vi "Filter_On_Start.vi"(10 "Num In":dbl[](array[numeric]), 11 "Denom In":dbl[](array[numeric])) -> (2 "Num out":dbl[](array[numeric]), 3 "Denom Out":dbl[](array[numeric]))   [LabVIEW 2014]
uses:
  Start.vi
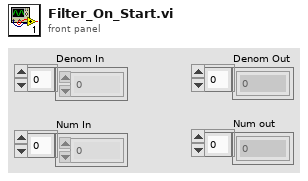
[diagram p1: front panel]
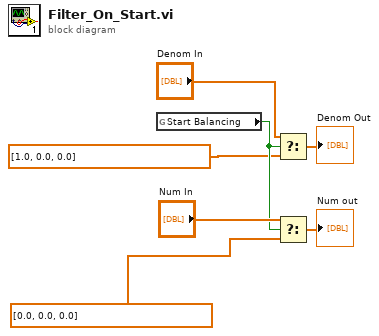
[diagram p0: block diagram]
diagram:
  n1 = global read "Start.vi" "Start Balancing"() -> (w6:bool)
  n2 = Select(t="Denom In", s=w6, f=dbl[] [1.0, 0.0, 0.0] ("Num Outer Loop")) -> (s? t:f=→"Denom Out":dbl[])
  n3 = Select(t="Num In", s=w6, f=dbl[] [0.0, 0.0, 0.0] ("Num Outer Loop")) -> (s? t:f=→"Num out":dbl[])
